vi "recordVideo.vi"() -> ()   [LabVIEW 2025]
panel:
  out "CPUorGPU":i32
  out "deviceNum":i32
  out "ExtrFramSucc":i32
  in  "noofFrames":u32=100
  in  "FramesPath":path=path "D:/labviewTestTCVdll/AnomalyDetection-LabVIEW/testFolder"
  out "success":i32
  out "resulting string":string
  in  "Path":path=path "D:/labviewTestTCVdll/AnomalyDetection-LabVIEW/recodedVideo"
  in  "duration(S)":u32=5
  in  "fps":u32=30
  in  "h":u32=720
  in  "w":u32=1280
  in  "cameraIndex":u32
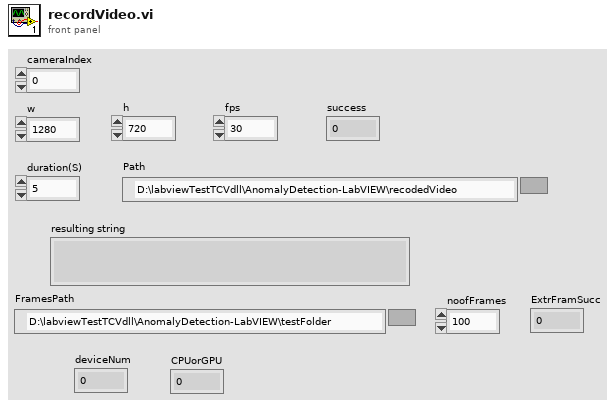
[diagram p1: front panel]
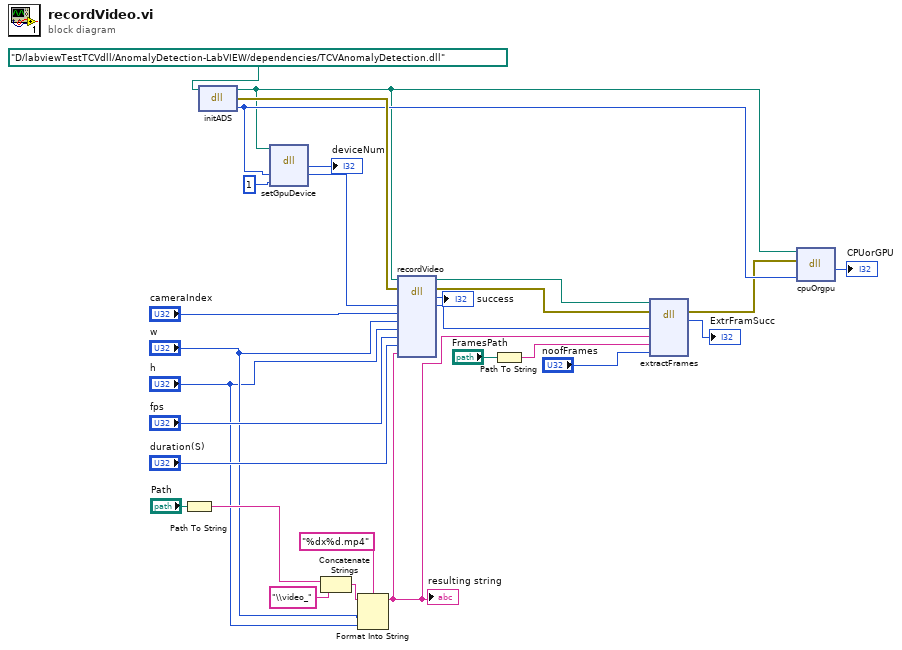
[diagram p0: block diagram]
diagram:
  n1 = Path To String(path="Path") -> (string=w26:string)
  n2 = dll-call lib="D:/labviewTestTCVdll/AnomalyDetection-LabVIEW/dependencies/AnomalyDetectionDLL.dll" fn="initADS"(path in=path "D:/labviewTestTCVdll/AnomalyDetection-LabVIEW/dependencies/TCVAnomalyDetection.dll") -> (path out=w9:path, error out=w15:errorcluster, "AnomalyDetectionInit"=w12:u64)  [unwired: 2 in]
  n3 = dll-call lib="D:/labviewTestTCVdll/AnomalyDetection-LabVIEW/dependencies/TCVAnomalyDetection.dll" fn="setGpuDevice"(path in=w9, "ref"=w12, "gpuNum"=u32 1) -> ("deviceNum"=→"deviceNum":i32, "ref"=w11:u64)  [unwired: 3 in, 2 out]
  n4 = Concatenate Strings(w26, "\\video_" ("string")) -> (w25:string)
  n5 = Format Into String(format string="%dx%d.mp4", initial string=w25, "w", "h") -> (resulting string=w17:string)  [unwired: 1 in, 1 out]
  "resulting string" <- w17
  n6 = dll-call lib="?" fn="recordVideo"(path in=w9, error in=w15, "ref"=w11, "cameraIndex"="cameraIndex", "w"="w", "h"="h", "fps"="fps", "duration(S)"="duration(S)", "path"=w17) -> (path out=w6:path, error out=w5:errorcluster, "success"=→"success":i32, "ref"=w1:u64)  [unwired: 7 in]
  n7 = Path To String(path="FramesPath") -> (string=w3:string)
  n8 = dll-call lib="?" fn="extractFrames"(path in=w6, error in=w5, "ref"=w1, "videoFile"=w17, "outputFolder"=w3, "noofFrames"="noofFrames") -> (error out=w10:errorcluster, "success"=→"ExtrFramSucc":i32)  [unwired: 5 in, 1 out]
  n9 = dll-call lib="D:/labviewTestTCVdll/AnomalyDetection-LabVIEW/dependencies/TCVAnomalyDetection.dll" fn="cpuOrgpu"(path in=w9, error in=w10, "ref"=w12) -> ("CPUorGPU"=→"CPUorGPU":i32)  [unwired: 2 in, 2 out]
